vi "Simulate iRobot Sensors.vi"(5 "accel smoothing (0-1)":dbl=0.1, 6 "Play Button":bool, 7 "Wheel Speed (mm/s)":i16(slide)=100 scale=0.0..500.0, 8 "error in":errorcluster, 11 "Cal Climber":T11) -> (0 "error out":errorcluster, 2 "Statechart Inputs":T1={"net distance (mm)"=0, "net angle (deg)"=0, "Max Wheel Speed (mm/s)"=0, "accelerometer"={"x axis (g)"=0.0, "y axis (g)"=0.0, "z axis (g)"=0.0}, "iRobot Sensors"={"Bumps + Wheel Drops"={"Wheeldrop Caster"=FALSE, "Wheeldrop Left"=FALSE, "Wheeldrop Right"=FALSE, "Bump Left"=FALSE, "Bump Right"=FALSE}, "Wall"=FALSE, "Cliff Left"=FALSE, "Cliff Front Left"=FALSE, "Cliff Front Right"=FALSE, "Cliff Right"=FALSE, "Virtual Wall"=FALSE, "Low-Side Driver + Wheel Overcurrent"={"Low-Side Driver 0"=FALSE, "Low-Side Driver 1"=FALSE, "Low-Side Driver 2"=FALSE, "Left Wheel"=FALSE, "Right Wheel"=FALSE}, "Infrared"=255, "Buttons"={"Advance"=FALSE, "Play"=FALSE}, "Distance (mm)"=0, "Angle (deg)"=0, "Charging State"=enum."Not Charging", "Voltage (mV)"=0, "Current (mA)"=0, "Battery Temperature (deg C)"=0, "Battery Charge (mAh)"=0, "Battery Capacity (mAh)"=0, "Wall Signal (0-4095)"=0, "Cliff Left Signal (0-4095)"=0, "Cliff Front Left Signal (0-4095)"=0, "Cliff Front Right Signal (0-4095)"=0, "Cliff Right Signal (0-4095)"=0, "Cargo Bay Digital Inputs"={"Digital Input 0"=FALSE, "Digital Input 1"=FALSE, "Digital Input 2"=FALSE, "Digital Input 3"=FALSE, "Device Detect"=FALSE}, "Cargo Bay Analog Signal (0-1023)"=0, "Charging Sources Available"={"Internal Charger"=FALSE, "Home Base"=FALSE}, "OI Mode"=enum."Off", "Song Number"=0, "Song Playing"=FALSE, "Number of Stream Packets"=0, "Requested Velocity (mm/s)"=0, "Requested Radius (mm)"=0, "Requested Right Wheel Velocity (mm/s)"=0, "Requested Left Wheel Velocity (mm/s)"=0}, "Is Simulator?"=FALSE} {"iRobot Sensors"."Infrared" format="%02x"; "accelerometer"."z axis (g)" format="%.3f"; "accelerometer"."y axis (g)" format="%.3f"; "accelerometer"."x axis (g)" format="%.3f"; "Max Wheel Speed (mm/s)" scale=0.0..500.0}, 3 "Cal Climber":T11)   [LabVIEW 2013]
doc: "Simulates iRobot sensors. Automatically accumulates distance and angle."
uses:
  Simulate iRobot.ctl
  <instrlib>/DC Motor Controller/HAIOL/DC Motor Controller.lvclass
  iRobot Navigation State Machine.lvsc/Inputs.ctl
  Accelerometer.ctl
  iRobot/Sensor/Sensor Group 6.ctl
  iRobot/Sensor/Bumps + Wheel Drops.ctl
  iRobot/Sensor/Low-Side Driver + Wheel Overcurrent.ctl
  iRobot/Sensor/Buttons.ctl
  iRobot/Sensor/Charging State.ctl
  iRobot/Sensor/Cargo Bay Digital Inputs.ctl
  iRobot/Sensor/Charging Sources Available.ctl
  iRobot/Sensor/OI Mode.ctl
  <vilib>/Analysis/coordinate.llb/Angle Units.ctl
  <vilib>/Analysis/coordinate.llb/Wrap Angle (scalar).vi
  <vilib>/Analysis/coordinate.llb/2D Cartesian Coordinate Rotation (Scalar).vi
  <vilib>/Analysis/BLAS.llb/dnrm2 - Vector 2-Norm (DBL).vi
  <resource>/objmgr/LVODE.rc
  <vilib>/Analysis/NI_AALBLAS.lvlib
  <vilib>/robotics/Kinematics/NI_Kinematics.lvlib
  <vilib>/Analysis/NI_AAL_Angle.lvlib
  <vilib>/Analysis/NI_AALPro.lvlib
  iRobot Navigation State Machine.lvsc
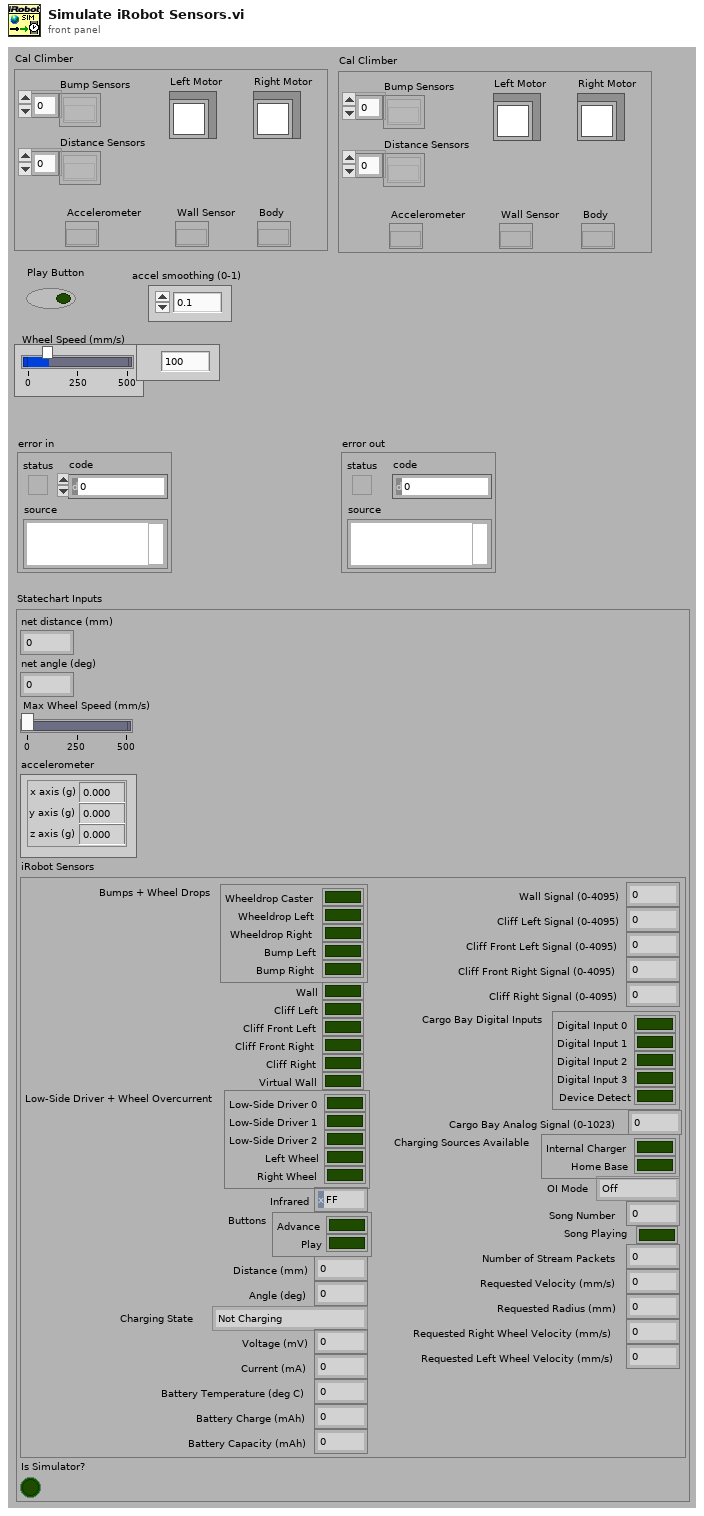
[diagram p1: front panel]
types:
  T1 = typedef "iRobot Navigation State Machine.lvsc/Inputs.ctl" = cluster{"net distance (mm)":i32, "net angle (deg)":i32, "Max Wheel Speed (mm/s)":i16, "accelerometer":T2, "iRobot Sensors":T3, "Is Simulator?":bool}
  T2 = typedef "Accelerometer.ctl" = cluster{"x axis (g)":dbl, "y axis (g)":dbl, "z axis (g)":dbl}
  T3 = typedef "Sensor Group 6.ctl" = cluster{"Bumps + Wheel Drops":T4, "Wall":bool, "Cliff Left":bool, "Cliff Front Left":bool, "Cliff Front Right":bool, "Cliff Right":bool, "Virtual Wall":bool, "Low-Side Driver + Wheel Overcurrent":T5, "Infrared":u8, "Buttons":T6, "Distance (mm)":i32, "Angle (deg)":i32, "Charging State":T7, "Voltage (mV)":u16, "Current (mA)":i16, "Battery Temperature (deg C)":i8, "Battery Charge (mAh)":u16, "Battery Capacity (mAh)":u16, "Wall Signal (0-4095)":u16, "Cliff Left Signal (0-4095)":u16, "Cliff Front Left Signal (0-4095)":u16, "Cliff Front Right Signal (0-4095)":u16, "Cliff Right Signal (0-4095)":u16, "Cargo Bay Digital Inputs":T8, "Cargo Bay Analog Signal (0-1023)":u16, "Charging Sources Available":T9, "OI Mode":T10, "Song Number":u8, "Song Playing":bool, "Number of Stream Packets":u8, "Requested Velocity (mm/s)":i16, "Requested Radius (mm)":i16, "Requested Right Wheel Velocity (mm/s)":i16, "Requested Left Wheel Velocity (mm/s)":i16}
  T4 = typedef "Bumps + Wheel Drops.ctl" = cluster{"Wheeldrop Caster":bool, "Wheeldrop Left":bool, "Wheeldrop Right":bool, "Bump Left":bool, "Bump Right":bool}
  T5 = typedef "Low-Side Driver + Wheel Overcurrent.ctl" = cluster{"Low-Side Driver 0":bool, "Low-Side Driver 1":bool, "Low-Side Driver 2":bool, "Left Wheel":bool, "Right Wheel":bool}
  T6 = typedef "Buttons.ctl" = cluster{"Advance":bool, "Play":bool}
  T7 = typedef "Charging State.ctl" = enum16{"Not Charging", "Reconditioning Charging", "Full Charging", "Trickle Charging", "Waiting", "Charging Fault Condition"}
  T8 = typedef "Cargo Bay Digital Inputs.ctl" = cluster{"Digital Input 0":bool, "Digital Input 1":bool, "Digital Input 2":bool, "Digital Input 3":bool, "Device Detect":bool}
  T9 = typedef "Charging Sources Available.ctl" = cluster{"Internal Charger":bool, "Home Base":bool}
  T10 = typedef "OI Mode.ctl" = enum16{"Off", "Passive", "Safe", "Full"}
  T11 = typedef "Simulate iRobot.ctl" = cluster{"Bump Sensors":refnum<k20>[], "Distance Sensors":refnum<k20>[], "Accelerometer":refnum<k20>, "Wall Sensor":refnum<k20>, "Body":refnum<k20>, "Left Motor":refnum<class "DC Motor Controller.lvclass">, "Right Motor":refnum<class "DC Motor Controller.lvclass">}
  T12 = typedef "NI_AAL_Angle.lvlib/Angle Units.ctl" = i32
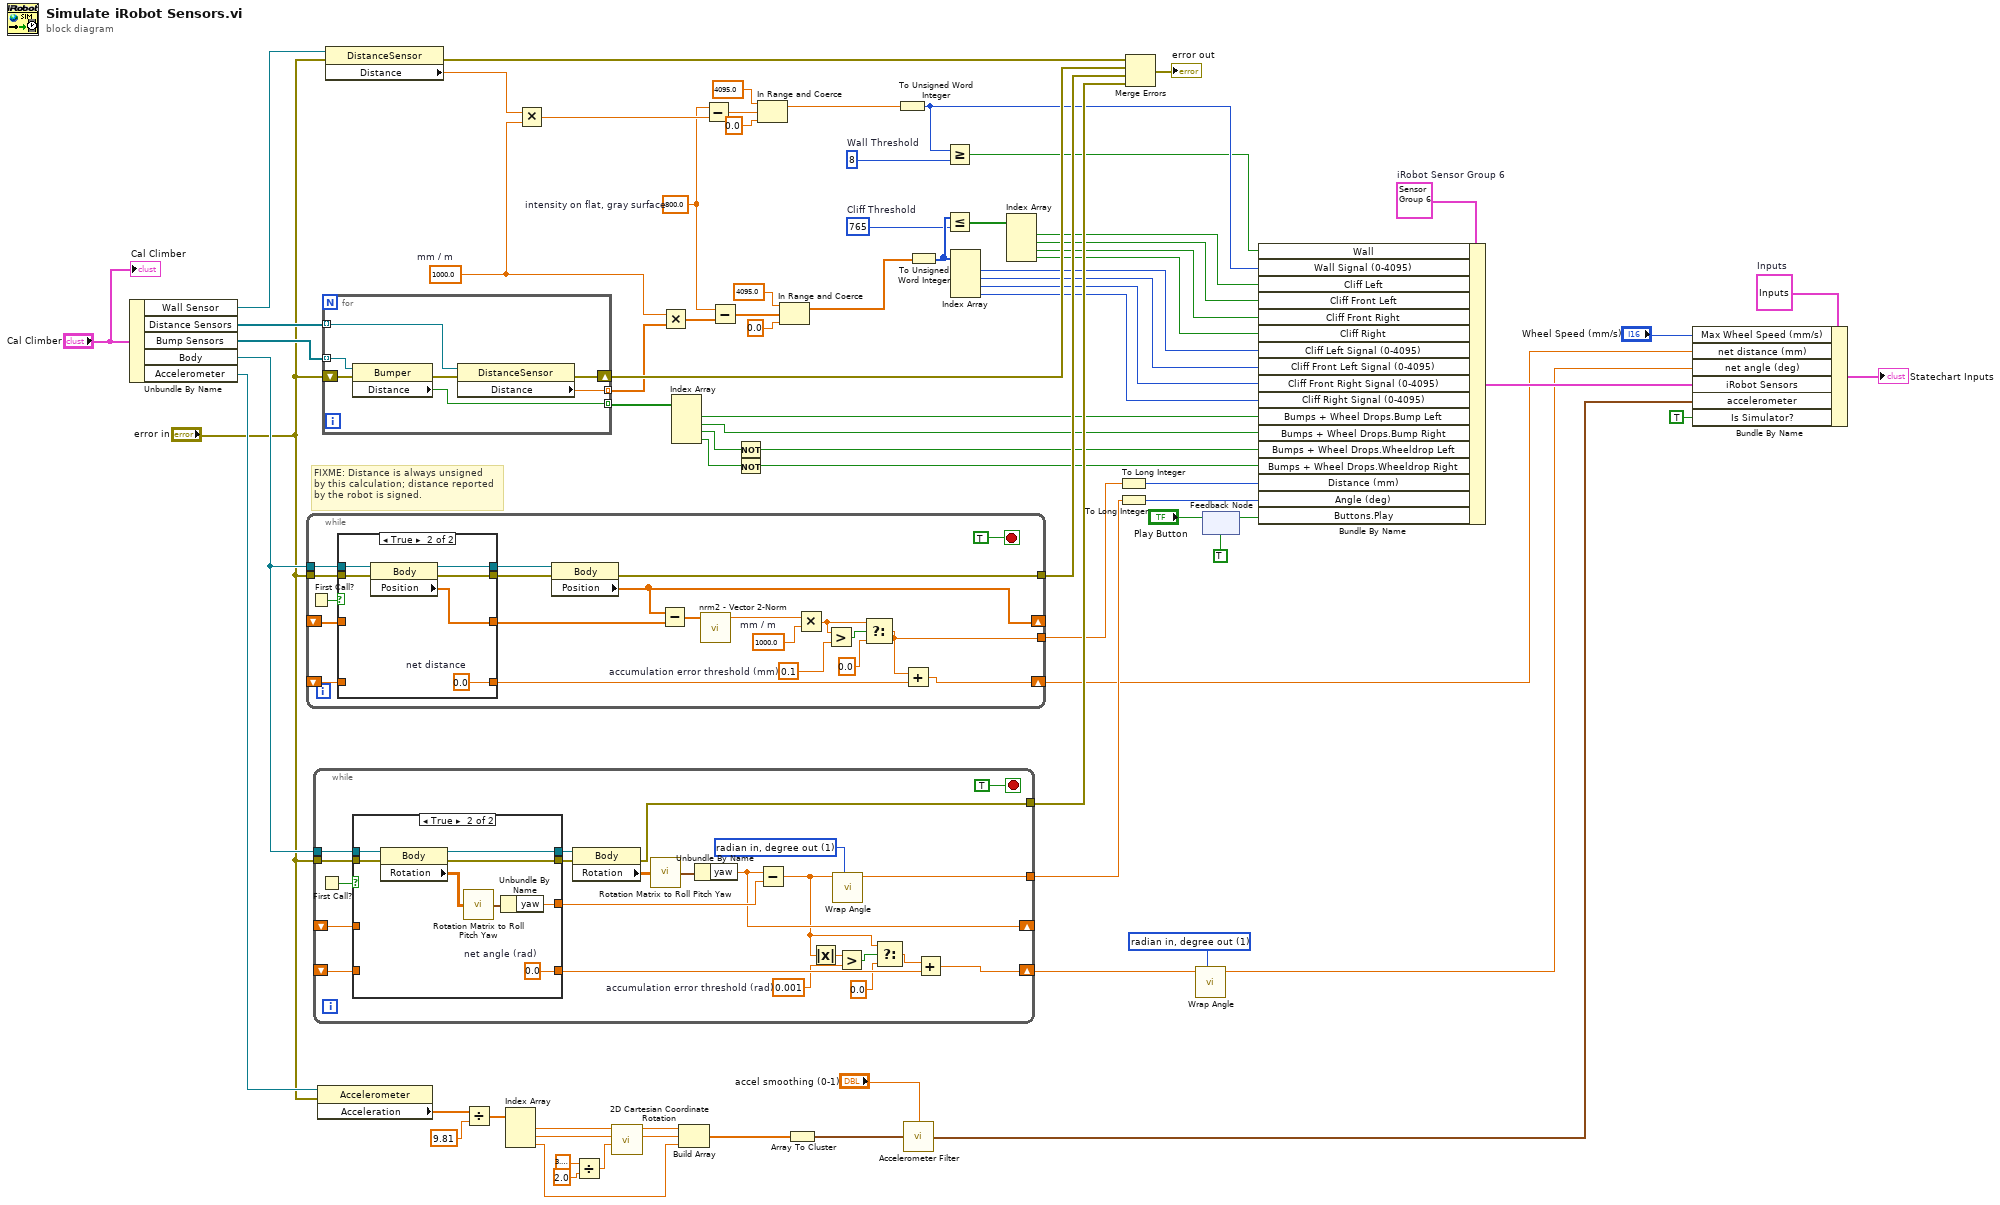
[diagram p0: block diagram]
diagram:
  w3 = T1 {"net distance (mm)"=0, "net angle (deg)"=0, "Max Wheel Speed (mm/s)"=0, "accelerometer"={"x axis (g)"=0.0, "y axis (g)"=0.0, "z axis (g)"=0.0}, "iRobot Sensors"={"Bumps + Wheel Drops"={"Wheeldrop Caster"=FALSE, "Wheeldrop Left"=FALSE, "Wheeldrop Right"=FALSE, "Bump Left"=FALSE, "Bump Right"=FALSE}, "Wall"=FALSE, "Cliff Left"=FALSE, "Cliff Front Left"=FALSE, "Cliff Front Right"=FALSE, "Cliff Right"=FALSE, "Virtual Wall"=FALSE, "Low-Side Driver + Wheel Overcurrent"={"Low-Side Driver 0"=FALSE, "Low-Side Driver 1"=FALSE, "Low-Side Driver 2"=FALSE, "Left Wheel"=FALSE, "Right Wheel"=FALSE}, "Infrared"=255, "Buttons"={"Advance"=FALSE, "Play"=FALSE}, "Distance (mm)"=0, "Angle (deg)"=0, "Charging State"=enum."Not Charging", "Voltage (mV)"=0, "Current (mA)"=0, "Battery Temperature (deg C)"=0, "Battery Charge (mAh)"=0, "Battery Capacity (mAh)"=0, "Wall Signal (0-4095)"=0, "Cliff Left Signal (0-4095)"=0, "Cliff Front Left Signal (0-4095)"=0, "Cliff Front Right Signal (0-4095)"=0, "Cliff Right Signal (0-4095)"=0, "Cargo Bay Digital Inputs"={"Digital Input 0"=FALSE, "Digital Input 1"=FALSE, "Digital Input 2"=FALSE, "Digital Input 3"=FALSE, "Device Detect"=FALSE}, "Cargo Bay Analog Signal (0-1023)"=0, "Charging Sources Available"={"Internal Charger"=FALSE, "Home Base"=FALSE}, "OI Mode"=enum."Off", "Song Number"=0, "Song Playing"=FALSE, "Number of Stream Packets"=0, "Requested Velocity (mm/s)"=0, "Requested Radius (mm)"=0, "Requested Right Wheel Velocity (mm/s)"=0, "Requested Left Wheel Velocity (mm/s)"=0}, "Is Simulator?"=FALSE}  # Inputs
  w37 = u16 8  # Wall Threshold
  w38 = 800.0  # intensity on flat, gray surface
  w42 = T12 1 items=["radian in, radian out", "radian in, degree out", "degree in, degree out", "degree in, radian out"] ("angle units")
  w46 = 765  # Cliff Threshold
  w66 = T3 {"Bumps + Wheel Drops"={"Wheeldrop Caster"=FALSE, "Wheeldrop Left"=FALSE, "Wheeldrop Right"=FALSE, "Bump Left"=FALSE, "Bump Right"=FALSE}, "Wall"=FALSE, "Cliff Left"=FALSE, "Cliff Front Left"=FALSE, "Cliff Front Right"=FALSE, "Cliff Right"=FALSE, "Virtual Wall"=FALSE, "Low-Side Driver + Wheel Overcurrent"={"Low-Side Driver 0"=FALSE, "Low-Side Driver 1"=FALSE, "Low-Side Driver 2"=FALSE, "Left Wheel"=FALSE, "Right Wheel"=FALSE}, "Infrared"=255, "Buttons"={"Advance"=FALSE, "Play"=FALSE}, "Distance (mm)"=0, "Angle (deg)"=0, "Charging State"=enum."Not Charging", "Voltage (mV)"=0, "Current (mA)"=0, "Battery Temperature (deg C)"=0, "Battery Charge (mAh)"=0, "Battery Capacity (mAh)"=0, "Wall Signal (0-4095)"=0, "Cliff Left Signal (0-4095)"=0, "Cliff Front Left Signal (0-4095)"=0, "Cliff Front Right Signal (0-4095)"=0, "Cliff Right Signal (0-4095)"=0, "Cargo Bay Digital Inputs"={"Digital Input 0"=FALSE, "Digital Input 1"=FALSE, "Digital Input 2"=FALSE, "Digital Input 3"=FALSE, "Device Detect"=FALSE}, "Cargo Bay Analog Signal (0-1023)"=0, "Charging Sources Available"={"Internal Charger"=FALSE, "Home Base"=FALSE}, "OI Mode"=enum."Off", "Song Number"=0, "Song Playing"=FALSE, "Number of Stream Packets"=0, "Requested Velocity (mm/s)"=0, "Requested Radius (mm)"=0, "Requested Right Wheel Velocity (mm/s)"=0, "Requested Left Wheel Velocity (mm/s)"=0}  # iRobot Sensor Group 6
  w72 = 1000.0  # mm / m
  # "FIXME: Distance is always unsigned\nby this calculation; distance reported\nby the robot is signed."
  n1 = Unbundle By Name("Cal Climber") -> ("Wall Sensor"=w77:refnum<k20>, "Distance Sensors"=w78:refnum<k20>[], "Bump Sensors"=w79:refnum<k20>[], "Body"=w41:refnum<k20>, "Accelerometer"=w28:refnum<k20>)
  n2 = while {
    tunnel: w41 -> [w100]
    tunnel: "error in" -> [w99]
    shift-right: [w87] -> _
    shift-left: _ -> [w97]
    tunnel: [w93] -> w69
    shift-right: [w88] -> w9
    shift-left: _ -> [w86]
    tunnel: [w80] -> w55
    stop <- TRUE stop-if-true
    w82 = 0.1  # accumulation error threshold (mm)
    w90 = 1000.0  # mm / m
    n3 = First Call?() -> (First Call?: T/F=w98:bool)
    n4 = case shown="True" w98 {
      tunnel: w100 -> [w102 w110]
      tunnel: w99 -> [w103 w109]
      tunnel: [w104 w106] -> w92
      tunnel: w97 -> [w104 _]
      tunnel: [w103 w108] -> w94
      tunnel: [w102 w107] -> w95
      tunnel: w86 -> [w101 _]
      tunnel: [w101 w105] -> w85
      frame False {
      }
      frame True {
        w105 = 0.0  # net distance
        n5 = property class="Body"(reference=w110, error in=w109) -> (reference out=w107:refnum<k20>, error out=w108:errorcluster, "Position"=w106:sgl[])
      }
    }
    n6 = property class="Body"(reference=w95, error in=w94) -> (error out=w93:errorcluster, "Position"=w87:sgl[])  [unwired: 1 out]
    n7 = Subtract(x=w87, y=w92) -> (x-y=w89:sgl[])
    n8 = call-poly <vilib>:"nrm2 - Vector 2-Norm.vi"("x"=w89) -> ("dnrm2"=w91:dbl)  [unwired: 9 in, 1 out]
    n9 = Multiply(x=w91, y=w90) -> (x*y=w84:dbl)
    n10 = Greater?(x=w84, y=w82) -> (0:w83:bool)
    n11 = Select(t=w84, s=w83, f=0.0) -> (s? t:f=w80:dbl)
    n12 = Add(x=w80, y=w85) -> (x+y=w88:dbl)
  }
  n13 = while {
    tunnel: w41 -> [w131]
    tunnel: "error in" -> [w130]
    tunnel: [w124] -> w68
    tunnel: [w111] -> w53
    shift-right: [w114] -> _
    shift-left: _ -> [w123]
    shift-right: [w121] -> w43
    shift-left: _ -> [w122]
    stop <- TRUE stop-if-true
    w112 = T12 1 items=["radian in, radian out", "radian in, degree out", "degree in, degree out", "degree in, radian out"] ("angle units")
    w116 = 0.001  # accumulation error threshold (rad)
    n14 = First Call?() -> (First Call?: T/F=w132:bool)
    n15 = case shown="True" w132 {
      tunnel: w131 -> [w137 w145]
      tunnel: w130 -> [w136 w144]
      tunnel: [w137 w143] -> w129
      tunnel: [w136 w142] -> w128
      tunnel: [w135 w139] -> w125
      tunnel: w123 -> [w135 _]
      tunnel: [w134 w138] -> w118
      tunnel: w122 -> [w134 _]
      frame False {
      }
      frame True {
        w138 = 0.0  # net angle (rad)
        n16 = property class="Body"(reference=w145, error in=w144) -> (reference out=w143:refnum<k20>, error out=w142:errorcluster, "Rotation"=w141:sgl[][])
        n17 = call <vilib>:"Rotation Matrix to Roll Pitch Yaw.vi"("rotation matrix"=w141) -> ("angles"=w140:cluster{"roll":dbl, "pitch":dbl, "yaw":dbl})
        n18 = Unbundle By Name(w140) -> ("yaw"=w139:dbl)
      }
    }
    n19 = property class="Body"(reference=w129, error in=w128) -> (error out=w124:errorcluster, "Rotation"=w127:sgl[][])  [unwired: 1 out]
    n20 = call <vilib>:"Rotation Matrix to Roll Pitch Yaw.vi"("rotation matrix"=w127) -> ("angles"=w126:cluster{"roll":dbl, "pitch":dbl, "yaw":dbl})
    n21 = Unbundle By Name(w126) -> ("yaw"=w114:dbl)
    n22 = Subtract(x=w114, y=w125) -> (x-y=w113:dbl)
    n23 = Absolute Value(x=w113) -> (abs(x)=w115:dbl)
    n24 = call-poly <vilib>:"Wrap Angle.vi"("angle units"=w112, "angle in"=w113) -> ("angle out"=w111:dbl)  [unwired: 8 in, 1 out]
    n25 = Greater?(x=w115, y=w116) -> (0:w120:bool)
    n26 = Select(t=w113, s=w120, f=0.0) -> (s? t:f=w119:dbl)
    n27 = Add(x=w119, y=w118) -> (x+y=w121:dbl)
  }
  n28 = property class="Accelerometer"(reference=w28, error in="error in") -> ("Acceleration"=w26:sgl[])  [unwired: 2 out]
  n29 = for {
    tunnel: [w152] -> w61 mode=indexing
    tunnel: w79 -> [w151] mode=indexing
    tunnel: [w150] -> w73 mode=indexing
    shift-right: [w147] -> w70
    shift-left: "error in" -> [w149]
    tunnel: w78 -> [w146] mode=indexing
    n30 = property class="Bumper"(reference=w151, error in=w149) -> (error out=w148:errorcluster, "Distance"=w150:bool)  [unwired: 1 out]
    n31 = property class="DistanceSensor"(reference=w146, error in=w148) -> (error out=w147:errorcluster, "Distance"=w152:sgl)  [unwired: 1 out]
  }
  n32 = property class="DistanceSensor"(reference=w77, error in="error in") -> (error out=w71:errorcluster, "Distance"=w76:sgl)  [unwired: 1 out]
  n33 = Divide(x=w26, y=9.81) -> (x/y=w23:dbl[])
  n34 = Index Array(array=w23) -> (element #1=w22:dbl, element #2=w21:dbl, element #3=w15:dbl)  [unwired: 3 in]
  n35 = Multiply(x=w76, y=w72) -> (x*y=w39:dbl)
  n36 = Divide(x=3.141592653589793, y=2.0) -> (x/y=w18:dbl)
  n37 = call-poly <vilib>:"2D Cartesian Coordinate Rotation.vi"("theta"=w18, "y"=w21, "x"=w22) -> ("y out"=w16:dbl, "x out"=w17:dbl)  [unwired: 6 in, 1 out]
  n38 = Multiply(x=w72, y=w61) -> (x*y=w40:dbl[])
  n39 = Index Array(array=w73) -> (element #1=w65:bool, element #2=w64:bool, element #3=w75:bool, element #4=w74:bool)  [unwired: 4 in]
  n40 = Build Array(w17, w16, w15) -> (w14:dbl[])
  n41 = Subtract(x=w38, y=w39) -> (x-y=w36:dbl)
  n42 = Subtract(x=w38, y=w40) -> (x-y=w30:dbl[])
  n43 = Not(x=w75) -> (.not. x?=w63:bool)
  n44 = Not(x=w74) -> (.not. x?=w62:bool)
  n45 = In Range and Coerce(upper limit=4095.0, x=w36, lower limit=0.0) -> (coerced(x)=w33:dbl)  [unwired: 1 out]
  n46 = In Range and Coerce(upper limit=4095.0, x=w30, lower limit=0.0) -> (coerced(x)=w29:dbl[])  [unwired: 1 out]
  n47 = Array To Cluster(array=w14) -> (cluster=w6:cluster{"[0]":dbl, "[1]":dbl, "[2]":dbl})
  n48 = To Unsigned Word Integer(number=w33) -> (unsigned 16bit integer=w45:u16)
  n49 = call "Accelerometer Filter.vi"("smoothing factor (0-1)"="accel smoothing (0-1)", "accelerometer (g)"=w6) -> ("filtered accelerometer (g)"=w4:T2)  [unwired: 2 in]
  n50 = To Unsigned Word Integer(number=w29) -> (unsigned 16bit integer=w52:u16[])
  n51 = Greater Or Equal?(x=w45, y=w37) -> (x >= y?=w44:bool)
  n52 = Less Or Equal?(x=w52, y=w46) -> (x <= y?=w51:bool[])
  n53 = Index Array(array=w52) -> (element #1=w60:u16, element #2=w59:u16, element #3=w58:u16, element #4=w57:u16)  [unwired: 4 in]
  n54 = Index Array(array=w51) -> (element #1=w47:bool, element #2=w48:bool, element #3=w49:bool, element #4=w50:bool)  [unwired: 4 in]
  n55 = To Long Integer(number=w55) -> (32bit integer=w56:i32)
  n56 = To Long Integer(number=w53) -> (32bit integer=w54:i32)
  n57 = Merge Errors(w71, w70, w69, w68) -> (→"error out":errorcluster)
  n58 = call-poly <vilib>:"Wrap Angle.vi"("angle units"=w42, "angle in"=w43) -> ("angle out"=w8:dbl)  [unwired: 8 in, 1 out]
  n59 = feedback-in #1("Play Button") -> ()
  n60 = feedback #1(TRUE) -> (w13:bool)
  n61 = Bundle By Name(cluster=w66, "Wall"=w44, "Wall Signal (0-4095)"=w45, "Cliff Left"=w47, "Cliff Front Left"=w48, "Cliff Front Right"=w49, "Cliff Right"=w50, "Cliff Left Signal (0-4095)"=w60, "Cliff Front Left Signal (0-4095)"=w59, "Cliff Front Right Signal (0-4095)"=w58, "Cliff Right Signal (0-4095)"=w57, "Bumps + Wheel Drops.Bump Left"=w65, "Bumps + Wheel Drops.Bump Right"=w64, "Bumps + Wheel Drops.Wheeldrop Left"=w63, "Bumps + Wheel Drops.Wheeldrop Right"=w62, "Distance (mm)"=w56, "Angle (deg)"=w54, "Buttons.Play"=w13) -> (w10:T3)
  n62 = Bundle By Name(cluster=w3, "Max Wheel Speed (mm/s)"="Wheel Speed (mm/s)", "net distance (mm)"=w9, "net angle (deg)"=w8, "iRobot Sensors"=w10, "accelerometer"=w4, "Is Simulator?"=TRUE) -> (→"Statechart Inputs":T1)
  "Cal Climber" <- "Cal Climber"
